vi "ReportTime.vi"(0 "Presence Vector":u8, 1 "Source":T1={"Subsystem Id"=3, "Node Id"=1, "Component Id"=1}, 2 "Destination":T1={"Subsystem Id"=90, "Node Id"=1, "Component Id"=1}, 3 "Time Stamp":timestamp=timestamp(3357882633.0878906 s since 1904-01-01), 5 "Sequence Number (16 bits)":u16=1) -> (7 "Encoded JAUS Message":string)   [LabVIEW 2009]
uses:
  Support Files/Address.ctl
panel:
  out "dateInt":u16
  out "timeInt":u32
  in  "Command Code":string="@\u0011"
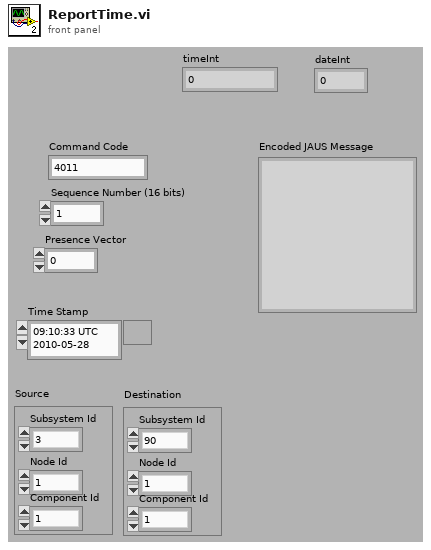
[diagram p1: front panel]
types:
  T1 = typedef "Address.ctl" = cluster{"Subsystem Id":u16, "Node Id":u8, "Component Id":u8}
  T2 = cluster{"unsigned byte array[0]":u8, "unsigned byte array[1]":u8}
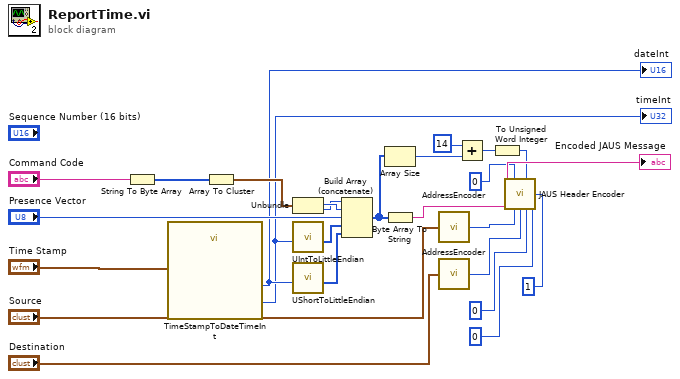
[diagram p0: block diagram]
diagram:
  n1 = String To Byte Array(string="Command Code") -> (unsigned byte array=w13:u8[])
  n2 = call "TimeStampToDateTimeInt.vi"("Time Stamp"="Time Stamp") -> ("timeInt"=w2:u32, "dateInt"=w3:u16)
  "timeInt" <- w2
  "dateInt" <- w3
  n3 = Array To Cluster(array=w13) -> (cluster=w12:T2)
  n4 = Unbundle(w12) -> ("unsigned byte array[0]"=w11:u8, "unsigned byte array[1]"=w10:u8)
  n5 = call "UIntToLittleEndian.vi"("Number"=w2) -> ("byte array"=w8:u8[])  [unwired: 10 in]
  n6 = call "UShortToLittleEndian.vi"("Number"=w3) -> ("byte array"=w7:u8[])  [unwired: 10 in]
  n7 = Build Array (concatenate)(w10, w11, "Presence Vector", w8, w7) -> (w17:u8[])
  n8 = Array Size(array=w17) -> (size(s)=w15:i32)
  n9 = Byte Array To String(unsigned byte array=w17) -> (string=w19:string)
  n10 = call "AddressEncoder.vi"("Address Cluster"="Source") -> ("Address"=w25:u32)
  n11 = call "AddressEncoder.vi"("Address Cluster"="Destination") -> ("Address"=w24:u32)
  n12 = Add(x=14, y=w15) -> (x+y=w14:i32)
  n13 = To Unsigned Word Integer(number=w14) -> (unsigned 16bit integer=w1:u16)
  n14 = call "JAUS Header Encoder.vi"("Message Type (0-5)"=u8 0, "Data Size (8-23)"=w1, "Priority(40-41)"=u8 1, "Payload"=w19, "Source ID (80-95)"=w25, "Destination ID (48-79)"=w24, "Data Flags (46-47)"=u8 0, "Ack/Nak (44-45)"=u8 0) -> ("Encoded JAUS Message"=→"Encoded JAUS Message":string)  [unwired: 7 in]
